vi "Write OffensivePlayRef.vi"(8 "error in (no error)":errorcluster, 10 "OffensivePlay":refnum<class "OffensivePlay.lvclass">, 11 "Team in":refnum<class "Team.lvclass">) -> (0 "error out":errorcluster, 3 "Team out":refnum<class "Team.lvclass">)   [LabVIEW 2018, in "Team.lvclass"]
uses:
  Team.lvclass
  OffensivePlay_class/OffensivePlay.lvclass
  Team.lvclass/Team.ctl
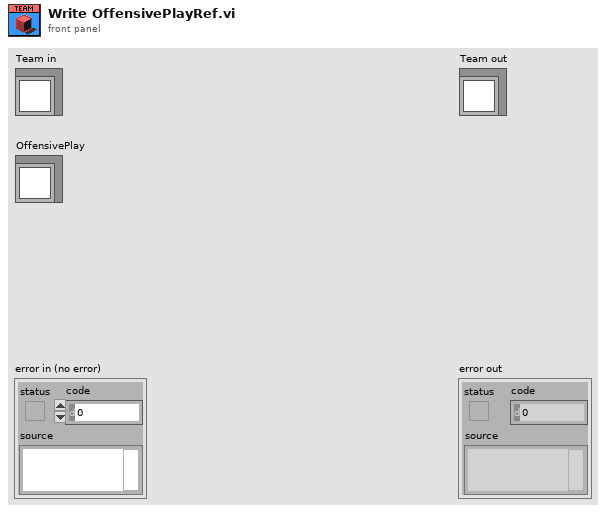
[diagram p1: front panel]
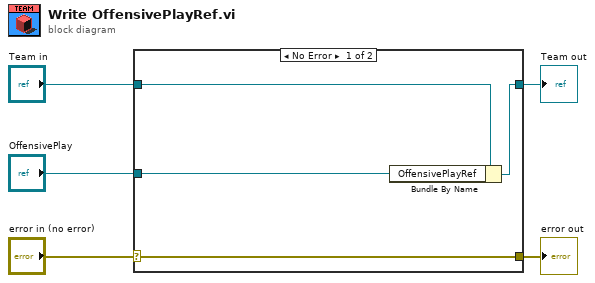
[diagram p0: block diagram]
diagram:
  n1 = case shown="No Error" "error in (no error)" {
    selector: "error in (no error)" -> [w9 w10]
    tunnel: [w9 w10] -> w4
    tunnel: [w7 w11] -> w2
    tunnel: "Team in" -> [w8 w11]
    tunnel: "OffensivePlay" -> [w6 _]
    frame No Error {
      n2 = Bundle By Name(cluster=w8, "OffensivePlayRef"=w6) -> (w7:refnum<class "Team.lvclass">)
    }
    frame Error {
    }
  }
  "error out" <- w4
  "Team out" <- w2
